vi "Draw xy.vi"(1 "Figur array":dbl[][](array[numeric]), 2 "Y":dbl, 3 "x":dbl) -> (0 "XY Graph":cluster{dbl[], dbl[]}[](graph))   [LabVIEW 2022 SP3]
panel:
  out "X array":dbl[](array[numeric])
  out "Y array":dbl[](array[numeric])
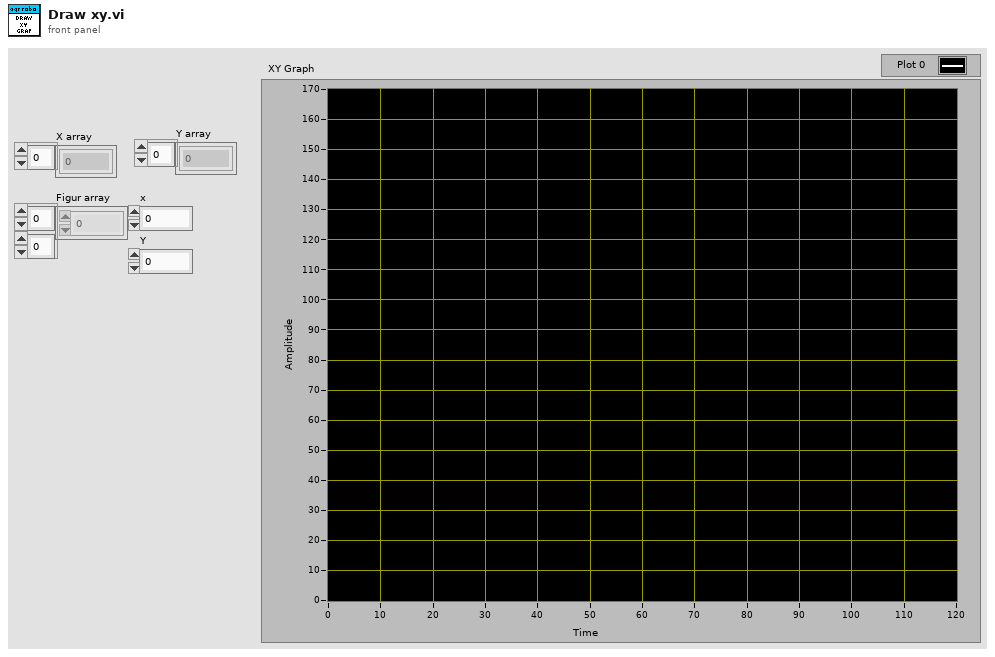
[diagram p1: front panel]
types:
  T1 = cluster{"Figur array":dbl[], "Figur array":dbl[]}
  T2 = cluster{"Figur array":dbl[], "Figur array":dbl[]}[]
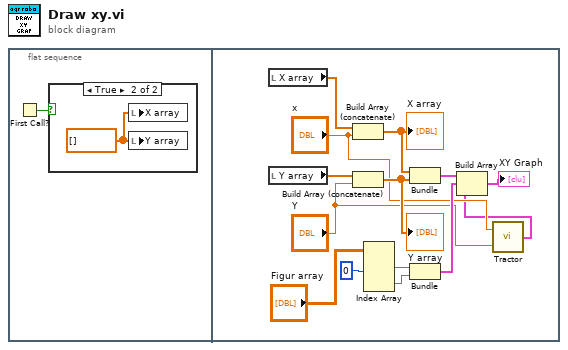
[diagram p0: block diagram]
diagram:
  n1 = flat-sequence {
    frame #0 {
      n2 = First Call?() -> (First Call?: T/F=w1:bool)
      n3 = case shown="True" w1 {
        frame False {
        }
        frame True {
          w2 = dbl[] [] ("X array")
          n4 = local write "X array"(w2) -> ()
          n5 = local write "Y array"(w2) -> ()
        }
      }
    }
    frame #1 {
      n6 = local read "X array"() -> (w6:dbl[])
      n7 = local read "Y array"() -> (w7:dbl[])
      n8 = Build Array (concatenate)(w6, "x") -> (w8:dbl[])
      "X array" <- w8
      n9 = Build Array (concatenate)(w7, "Y") -> (w9:dbl[])
      "Y array" <- w9
      n10 = Index Array(array="Figur array", index (col) #1=0 ("disabled index (col)")) -> (element #1=w14:dbl[], element #2=w15:dbl[])  [unwired: 3 in]
      n11 = Bundle(w8, w9) -> (w11:cluster{dbl[], dbl[]})  [unwired: 1 in]
      n12 = Bundle("Figur array"=w14, "Figur array"=w15) -> (w13:T1)  [unwired: 1 in]
      n13 = call "Tractor.vi"("Y"="Y", "X"="x") -> ("XY Graph"=w3:cluster{dbl[], dbl[]})
      n14 = Build Array(w11, w13, w3) -> (→"XY Graph":T2)
    }
  }
